vi "Copy Render to Clipboard.vi"(8 "error in":errorcluster, 11 "BigMAQ in":refnum<class "BigMAQ.lvclass">) -> (0 "error out":errorcluster, 3 "BigMAQ out":refnum<class "BigMAQ.lvclass">)   [LabVIEW 2019, in "BigMAQ.lvclass"]
uses:
  BigMAQ.lvclass
  <vilib>/LabVIEW Open Source Project/Unicity/RandomStringGenerator/RandomStringGenerator.lvclass
  <vilib>/vision/NI_Vision_Development_Module.lvlib
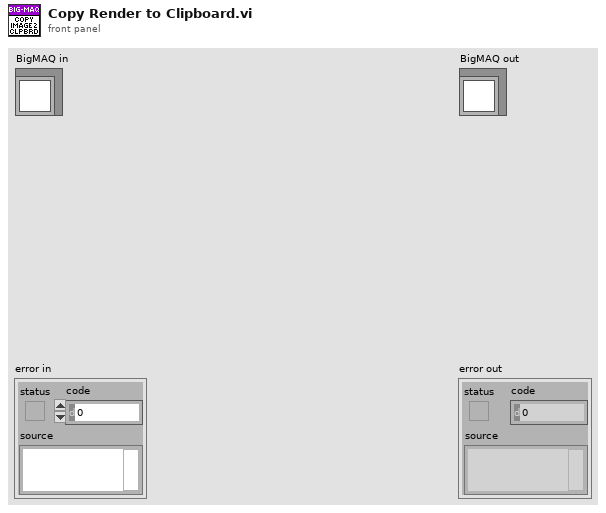
[diagram p1: front panel]
types:
  T1 = typedef "Image Type" = u32
  T2 = typedef "IMAQ Image.ctl" = refnum<image>
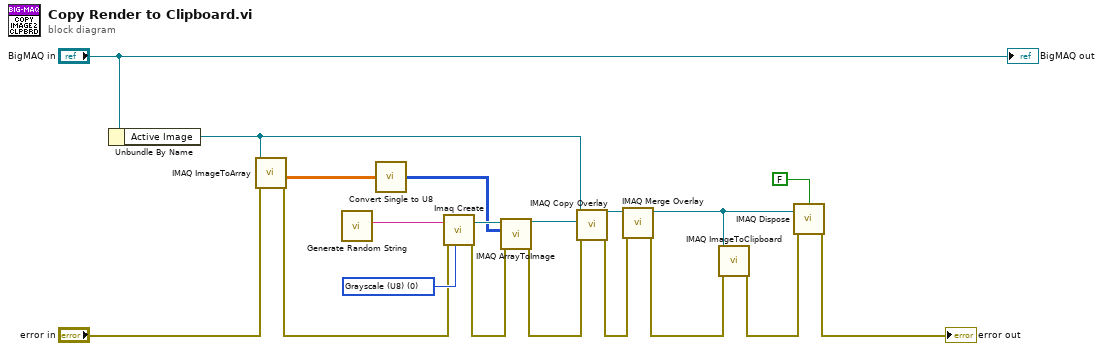
[diagram p0: block diagram]
diagram:
  w18 = T1 0 items=["Grayscale (U8)", "Grayscale (I16)", "Grayscale (SGL)", "Complex (CSG)", "RGB (U32)", "HSL (U32)", "RGB (U64)", "Grayscale (U16)"] ("Image Type")
  n1 = Unbundle By Name("BigMAQ in") -> ("Active Image"=w12:T2)
  n2 = call "IMAQ ImageToArray"("error in (no error)"="error in", "Image"=w12) -> ("Image Pixels (Float)"=w16:sgl[][], "error out"=w9:errorcluster)  [unwired: 2 in, 3 out]
  n3 = call <vilib>:"Generate Random String.vi"() -> ("Random String"=w11:string)  [unwired: 11 in]
  n4 = call "Convert Single to U8.vi"("Image Pixels (Float)"=w16) -> ("Image Pixels (U8)"=w15:u8[][])
  n5 = call "Imaq Create"("Image Name"=w11, "Image Type"=w18, "error in (no error)"=w9) -> ("New Image"=w17:T2, "error out"=w8:errorcluster)  [unwired: 2 in]
  n6 = call "IMAQ ArrayToImage"("error in (no error)"=w8, "Image Pixels (U8)"=w15, "Image"=w17) -> ("error out"=w7:errorcluster, "Image Out"=w13:T2)  [unwired: 7 in]
  n7 = call "IMAQ Copy Overlay"("error in (no error)"=w7, "Image Dst"=w13, "Image Src"=w12) -> ("error out"=w6:errorcluster, "Image Dst Out"=w14:T2)  [unwired: 7 in]
  n8 = call "IMAQ Merge Overlay"("error in (no error)"=w6, "Image Src"=w14) -> ("error out"=w2:errorcluster, "Image Dst Out"=w1:T2)  [unwired: 8 in]
  n9 = call "IMAQ ImageToClipboard"("Image"=w1, "error in (no error)"=w2) -> ("error out"=w3:errorcluster)  [unwired: 4 in]
  n10 = call "IMAQ Dispose"("All Images? (No)"=FALSE, "Image"=w1, "error in (no error)"=w3) -> ("error out"=→"error out":errorcluster)  [unwired: 3 in]
  "BigMAQ out" <- "BigMAQ in"
